vi "Read Datalog File.vi"(0 "Data Log File Refnum":refnum<k1>, 1 "number of acquisitions":i32=10) -> (2 "Array Data Out":cluster{string, "empty array":sgl[]}[](array[cluster]) {"empty array" format="%0.2f"}, 4 "error out":errorcluster)   [LabVIEW 2010]
doc: "Opens the datalog file created by the Write Datalog File Example VI in this LLB and reads one record at a time from the file until all are read. Each record is a cluster containing a timestamp string and an array of single-precision numbers."
panel:
  out "record data":sgl[](graph)
  out "record time":string
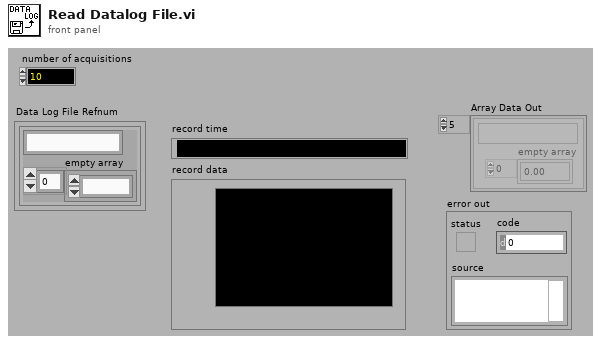
[diagram p1: front panel]
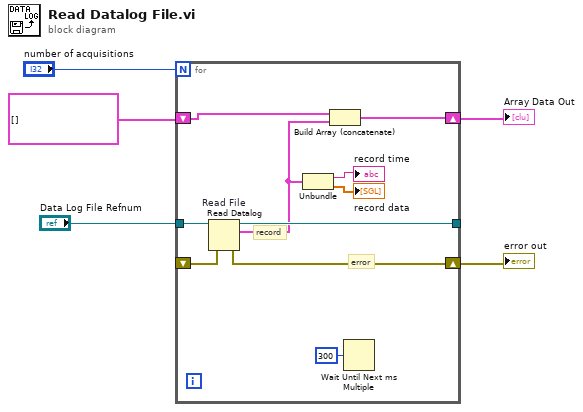
[diagram p0: block diagram]
diagram:
  n1 = for {
    N: "number of acquisitions" -> [_]
    tunnel: [w15] -> _
    tunnel: "Data Log File Refnum" -> [w14]
    shift-right: [w10] -> w2
    shift-left: cluster{string, "empty array":sgl[]}[] [] -> [w11]
    shift-right: [w7] -> w1
    shift-left: _ -> [w8]
    # "record"
    # "error"
    n2 = Read Datalog "Read File"(4:w8, 7:w14) -> (0:w7:errorcluster, 2:w9:cluster{string, "empty array":sgl[]}, 3:w15:refnum<k1>)  [unwired: 1 out]
    n3 = Unbundle(w9) -> (→"record time":string, "empty array"=→"record data":sgl[])
    n4 = Build Array (concatenate)(w11, w9) -> (w10:cluster{string, "empty array":sgl[]}[])
    n5 = Wait Until Next ms Multiple(millisecond multiple=u32 300) -> ()  [unwired: 1 out]
  }
  "error out" <- w1
  "Array Data Out" <- w2
